vi "add Tests.vi"(8 "error in (no error)":errorcluster caption="Fehler (Eingang, kein Fehler)", 10 "Tests":refnum<class "TestInterface.lvclass">[](array[class]), 11 "DeviceInterface (Eingang)":refnum<class "DeviceInterface.lvclass">) -> (0 "error out":errorcluster caption="Fehler (Ausgang)", 3 "DeviceInterface (Ausgang)":refnum<class "DeviceInterface.lvclass">)   [LabVIEW 2013, in "DeviceInterface.lvclass"]
uses:
  DeviceInterface.lvclass
  Tests/TestInterface/TestInterface.lvclass
  DeviceInterface.lvclass/DeviceInterface.ctl
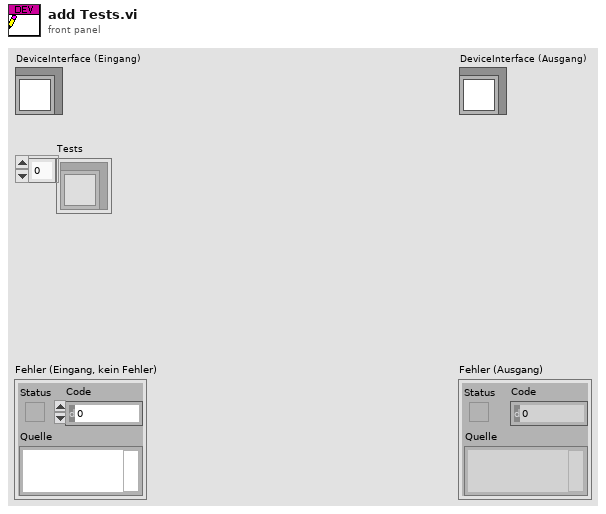
[diagram p1: front panel]
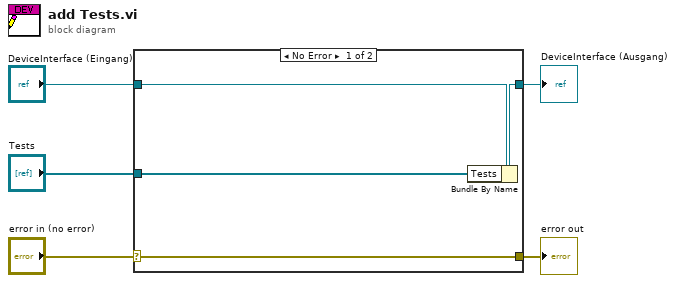
[diagram p0: block diagram]
diagram:
  n1 = case shown="No Error" "error in (no error)" {
    selector: "error in (no error)" -> [w9 w10]
    tunnel: [w9 w10] -> w4
    tunnel: [w7 w11] -> w2
    tunnel: "DeviceInterface (Eingang)" -> [w8 w11]
    tunnel: "Tests" -> [w6 _]
    frame No Error {
      n2 = Bundle By Name(cluster=w8, "Tests"=w6) -> (w7:refnum<class "DeviceInterface.lvclass">)
    }
    frame Error {
    }
  }
  "error out" <- w4
  "DeviceInterface (Ausgang)" <- w2
